vi "SubVI_Get2DTemperatureArray.vi"(9 "af1DTempMat":sgl[](array[numeric]), 11 "ErrorIn":errorcluster) -> (0 "i32Width":i32, 1 "i32Height":i32, 2 "af2DTempMat":sgl[][](array[numeric]), 3 "ErrorOut":errorcluster, 4 "u8Error":i32)   [LabVIEW 2013]
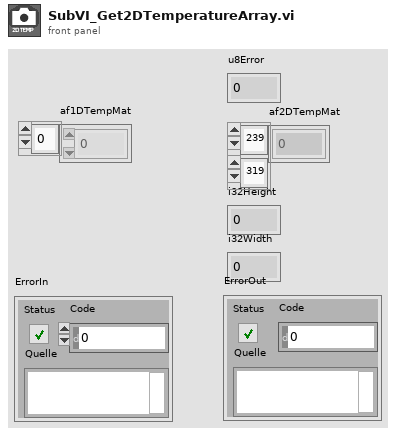
[diagram p1: front panel]
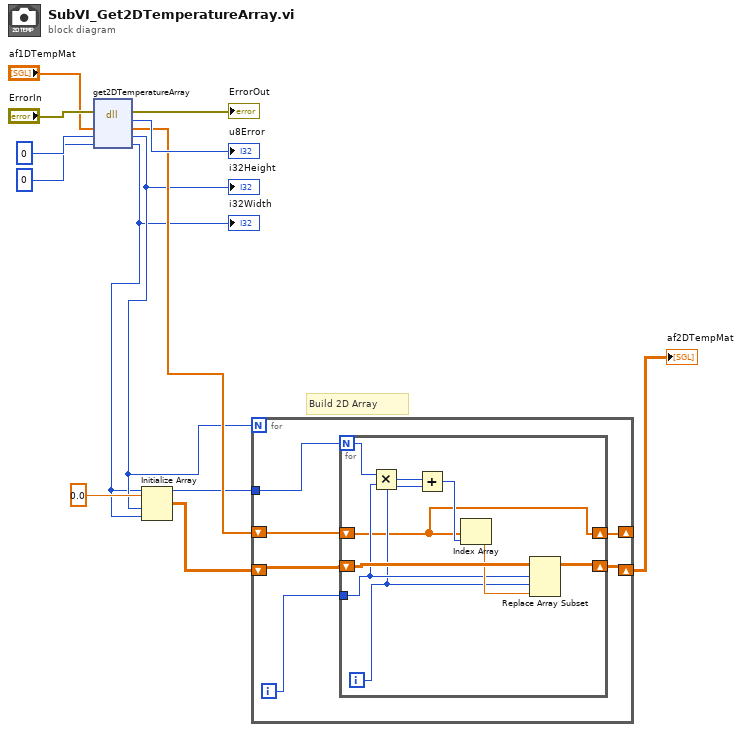
[diagram p0: block diagram]
diagram:
  # "Build 2D Array"
  n1 = dll-call lib="PTH1abs CUsers1000len-bimDesktop&Lieferung_LabView_Interface_11.11.2015Einrichten fÃ¼r - EndkundenDatenTesto_v2013VIlabview_cwrapper_1_0_0.dll" fn="get2DTemperatureArray"(error in="ErrorIn", "af2DTempMat"="af1DTempMat", "i32Height"=0, "i32Width"=0) -> (error out=→"ErrorOut":errorcluster, "u8Error"=→"u8Error":i32, "af2DTempMat"=w5:sgl[], "i32Height"=w4:i32, "i32Width"=w3:i32)  [unwired: 2 in, 1 out]
  "i32Height" <- w4
  "i32Width" <- w3
  n2 = Initialize Array(sgl 0.0 ("Element"), w4, w3) -> (w7:sgl[][])
  n3 = for {
    N: w4 -> [_]
    shift-right: [w17] -> w6
    shift-left: w7 -> [w18]
    tunnel: w3 -> [w15]
    shift-right: [w13] -> _
    shift-left: w5 -> [w14]
    i -> [w16]
    n4 = for {
      N: w15 -> [w24]
      shift-right: [w26] -> w17
      shift-left: w18 -> [w27]
      tunnel: w16 -> [w23]
      shift-right: [w19] -> w13
      shift-left: w14 -> [w19]
      i -> [w21]
      n5 = Multiply(x=w24, y=w23) -> (x*y=w22:i32)
      n6 = Add(x=w22, y=w21) -> (x+y=w20:i32)
      n7 = Index Array(array=w19, index=w20) -> (element=w25:sgl)
      n8 = Replace Array Subset(array=w27, new element=w25, index (row)=w23, index (col)=w21) -> (w26:sgl[][])
    }
  }
  "af2DTempMat" <- w6
